vi "Destroy Session.vi"(0 "reference in":refnum<class "J1939-22_Engine.lvclass">, 5 "Error In":errorcluster) -> (14 "reference out":refnum<class "J1939-22_Engine.lvclass">, 19 "Error Out":errorcluster)   [LabVIEW 2021, in "J1939-22_Engine.lvclass"]
uses:
  J1939-22_Engine.lvclass
  J1939-22_Engine.lvclass/J1939-22_Engine.ctl
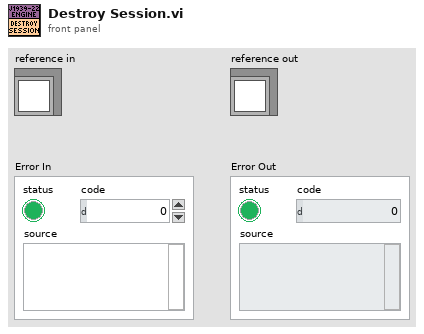
[diagram p1: front panel]
types:
  T1 = typedef "J1939-22_Engine.lvclass/ObjectAttributes.ctl" = cluster{"Data":T2[], "DTCs":T15[], "XNET.Settings.Database":refnum<k21>, "J1939-22_Database":refnum<class "J1939-22_Database.lvclass">}
  T2 = typedef "J1939 Addon Engine.lvlib/Protocol.XNET Refs.ctl" = cluster{"Network":T3, "Incoming.Use":bool, "Incoming.Session":refnum<k21>, "Incoming.Refs":T4[], "Incoming.Values":dbl[], "Outgoing.Frames":T6[], "Outgoing.Initialize":bool, "Outgoing.Refs":T4[], "Outgoing.Values":dbl[], "Request.Table":refnum<k33>, "Timing.Use":bool, "Timing.Index":i32[], "Timing.Refs":T4[], "Timing.Values":dbl[], "Disable.Refs":T4[], "Disable.Values":dbl[], "Trigger.Refs":T4[], "Trigger.Values":dbl[], "Outgoing.Frames.CountersAndProtections":T8[]}
  T3 = typedef "J1939 Addon Shared.lvlib/Monitor Settings.ctl" = cluster{"Address":u8, "Name":u64, "Include DA":bool, "Force SA":bool}
  T4 = typedef "Custom Device API.lvlib/Block Data Reference.ctl" = cluster{"Data Reference":T5, "Offset":u64, "Length":u64}
  T5 = typedef "Custom Device API.lvlib/Data Reference.ctl" = i32
  T6 = typedef "J1939 Addon Engine.lvlib/Main.Outgoing.Frame.Settings.ctl" = cluster{"Offset":u32, "Length":u32, "Cyclic":bool, "Disable.Index":i32, "Disable":bool, "Trigger":T7, "Trigger.Index":i32, "Session":refnum<k21>}
  T7 = typedef "J1939 Addon Shared.lvlib/Outgoing Event Trigger Types.ctl" = enum16{"Channel value change", "Trigger channel (not zero)", "Channel value change or trigger channel (not zero)", "Trigger channel (any value change)", "Channel value change or trigger channel (any value change)"}
  T8 = typedef "Protection and Counter Support Shared.lvlib/Exported Frame Settings.ctl" = cluster{"Type":T9, "Frame ID":u32, "Payload Length":u32, "Signal XNET Paths":string[], "Frame.PrevData":dbl[], "VS Offset":i32, "VS Length":i32, "Generation Period":u32, "Has Protection?":bool, "Protection Configurations":T10[], "Has Counter":bool, "Counter Configurations":T13[], "Has Disable?":bool, "Disable VS Index":i32, "Transmit Trigger":T14, "Trigger VS Index":i32}
  T9 = typedef "Protection and Counter Support Shared.lvlib/Exported Frame Type.ctl" = enum16{"Periodic", "Event", "Periodic/Event"}
  T10 = typedef "Protection and Counter Support Shared.lvlib/Exported Protection Settings.ctl" = cluster{"Protection Frame Index":i32, "Protection Type":T11, "Data Indeces":i32[], "Initialized Data Array":dbl[], "Protection Signal XNET Paths":string[], "CRC Channels":T12[], "Protection VS Update Index":i32, "Override Index":i32, "Override Value Index":i32}
  T11 = typedef "Protection and Counter Support Shared.lvlib/Protection Type.ctl" = enum16{"Arb ID + Bytes Checksum with Inversion", "Arb ID + Bytes CRC with Inversion", "Reversed Raw Signal Checksum with Inversion", "Concatenated Two's Compliment"}
  T12 = typedef "Protection and Counter Support Shared.lvlib/XNET Signal Configuration.ctl" = cluster{"Start Bit":i32, "Name":string, "Number of bits":i32, "Scale":dbl, "Offset":dbl, "Data Type":u32, "Counter":bool}
  T13 = typedef "Protection and Counter Support Shared.lvlib/Exported Counter Settings.ctl" = cluster{"Frame Index":i32, "Max Count":dbl, "VS Index":i32, "Bit Length":i64, "Override Index":i32, "Override Value Index":i32}
  T14 = typedef "Protection and Counter Support Shared.lvlib/Exported Event Trigger Type.ctl" = enum16{"Channel value change", "Trigger channel (not zero)", "Channel value change or trigger channel (not zero)", "Trigger channel (any value change)", "Channel value change or trigger channel (any value change)"}
  T15 = typedef "J1939 Addon Engine.lvlib/Engine.DTC Settings.ctl" = cluster{"Data":T16, "FIFOs":T17}
  T16 = typedef "J1939 Addon Shared.lvlib/Compiled Simulated Settings.ctl" = cluster{"DM1.Ref":T4[], "DM1.Value":dbl[], "DM1.Enable.Ref":T4[], "DM1.Enable.Value":dbl[], "DM2.Ref":T4[], "DM2.Value":dbl[], "DM2.Enable.Ref":T4[], "DM2.Enable.Value":dbl[]}
  T17 = typedef "J1939 Addon Engine.lvlib/Engine.DTC FIFOs.ctl" = cluster{"DM1.Data":refnum<k33>, "DM1.Enable":refnum<k33>, "DM2.Data":refnum<k33>, "DM2.Enable":refnum<k33>, "DM1.Reset":refnum<k33>, "DM2.Reset":refnum<k33>}
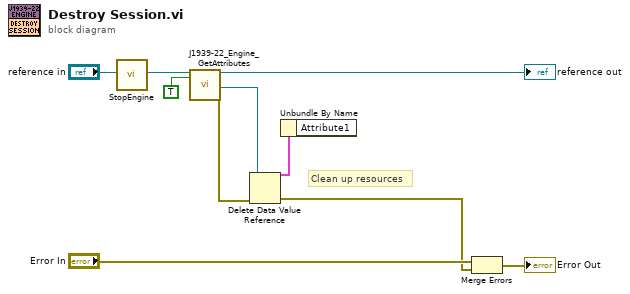
[diagram p0: block diagram]
diagram:
  # "Clean up resources"
  n1 = call "StopEngine.vi"("reference in"="reference in") -> ("reference out"=w1:refnum<class "J1939-22_Engine.lvclass">)  [unwired: 17 in, 1 out]
  n2 = call "J1939-22_Engine_GetAttributes.vi"("reference in"=w1, "OnlyGetDvrReference(False)"=TRUE) -> ("reference out"=→"reference out":refnum<class "J1939-22_Engine.lvclass">, "DataRef"=w7:refnum<data-value>, "Error Out"=w8:errorcluster)  [unwired: 14 in, 1 out]
  n3 = Delete Data Value Reference(data value reference=w7, error in=w8) -> (data value=w3:T1, error out=w5:errorcluster)
  n4 = Unbundle By Name(w3) -> ()  [unwired: 1 out]
  n5 = Merge Errors("Error In", w5) -> (→"Error Out":errorcluster)
